vi "rwr_getNextStepsToExecute.vi"(4 "Show in Debugger?":bool=TRUE, 6 "Message Priority":T1=enum."Normal", 7 "Caller in":refnum<class "Worker.lvclass">, 8 "error in":errorcluster, 9 "timeout (ms)":i32=5000, 11 "sequenceManagerWorker in":refnum<class "sequenceManagerWorker.lvclass">) -> (0 "error out":errorcluster, 2 "StepsToExecuteInParallel":refnum<class "Step.lvclass">[](array[class]), 3 "dup sequenceManagerWorker out":refnum<class "sequenceManagerWorker.lvclass">, 5 "dup Caller out":refnum<class "Worker.lvclass">)   [LabVIEW 2023, in "sequenceManagerWorker.lvclass"]
doc: "This VI sends a <b>Public API Request with Reply</b> message to an MHL case of the Worker that owns this VI. This VI will wait until it receives a <b>Reply</b> message back from the Worker that owns this VI. If the wait time exceeds <b>timeout (ms)</b>, an error will be returned.\n---\nThis request gets the next series of steps to execute in parallel."
uses:
  sequenceManagerWorker.lvclass
  <vilib>/addons/_Workers/Library/Classes/Worker/Worker.lvclass
  <vilib>/addons/_Workers/Library/Classes/Message/Priority.ctl
  ZE_Easy.Sequencer.lvlibp/Step/Step.lvclass
  rwr_getNexytStepsToExecute.ctl
  rwr_getNexytStepsToExecute Reply.ctl
  <vilib>/addons/_Workers/Library/Case Label.ctl
  <vilib>/addons/_Workers/Library/Classes/Message Queue/Message Queue.lvclass
  <vilib>/addons/_Workers/Library/Workers.lvlib
  <vilib>/addons/_Workers/Library/Classes/Message/Message.lvclass
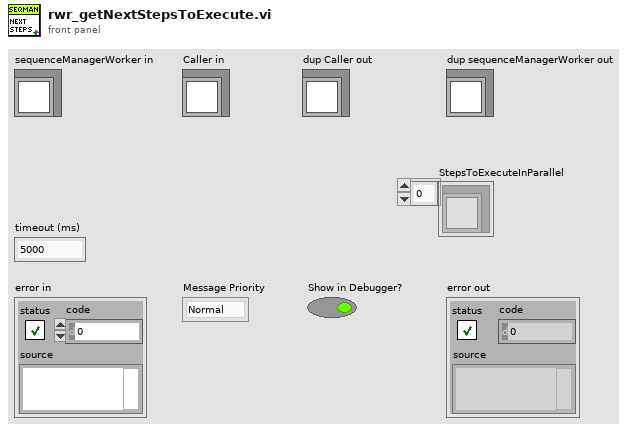
[diagram p1: front panel]
types:
  T1 = typedef "Workers.lvlib/Message.lvclass/Priority.ctl" = enum16{"Low", "Normal", "High"}
  T2 = typedef "sequenceManagerWorker.lvclass/rwr_getNexytStepsToExecute.ctl" = cluster{"String":string}
  T3 = typedef "sequenceManagerWorker.lvclass/rwr_getNexytStepsToExecute Reply.ctl" = cluster{"StepsToExecuteInParallel":refnum<class "Step.lvclass">[]}
  T4 = typedef "Workers.lvlib/Case Label.ctl" = string
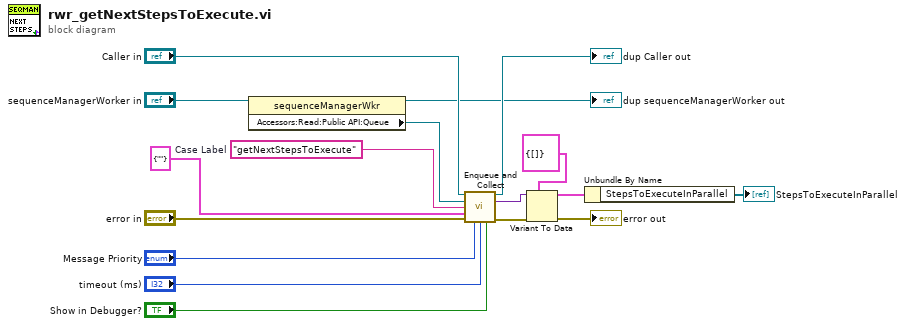
[diagram p0: block diagram]
diagram:
  w4 = T4 "getNextStepsToExecute"  # Case Label
  n1 = property class="sequenceManagerWkr"(reference="sequenceManagerWorker in") -> (reference out=→"dup sequenceManagerWorker out":refnum<class "sequenceManagerWorker.lvclass">, "Accessors:Read:Public API:Queue"=w5:refnum<class "Message Queue.lvclass">)  [unwired: 1 in, 1 out]
  n2 = call-dynamic "Enqueue and Collect.vi"("Worker"="Caller in", "Message Queue"=w5, "Case Label"=w4, "Data"=T2 {"String"=""} ("Data in"), "error in (no error)"="error in", "Priority (Normal)"="Message Priority", "timeout in ms"="timeout (ms)", "Send Message to Debugger? (T)"="Show in Debugger?") -> ("dup Worker out"=→"dup Caller out":refnum<class "Worker.lvclass">, "Data out"=w10:variant, "error out"=w11:errorcluster)  [unwired: 4 in, 1 out]
  n3 = Variant To Data(error in=w11, type=T3 {"StepsToExecuteInParallel"=[]} ("Reply Data out"), Variant=w10) -> (data=w2:T3, error out=→"error out":errorcluster)
  n4 = Unbundle By Name(w2) -> ("StepsToExecuteInParallel"=→"StepsToExecuteInParallel":refnum<class "Step.lvclass">[])
